vi "Add file.vi"(8 "error in (no error)":errorcluster, 9 "Insert in front":bool, 10 "File Path":path, 11 "MagLabGraph in":refnum<class "XY Plot.lvclass">) -> (0 "error out":errorcluster, 2 "Success":bool, 3 "MagLabGraph out":refnum<class "XY Plot.lvclass">)   [LabVIEW 2019, in "XY Plot.lvclass"]
uses:
  XY Plot.lvclass
  C:/Program Files/National Instruments/LabVIEW 2019/vi.lib/ActorFramework/Actor/Actor.lvclass
  C:/GitHub/LabActor/Plots/Plot/Plot.lvclass
  <vilib>/ActorFramework/Actor/Actor.lvclass/Actor.ctl
  <vilib>/ActorFramework/Message Enqueuer/Message Enqueuer.lvclass/Message Enqueuer.ctl
  Plot Messages/Add file Msg/Add file Msg.lvclass/Add file Msg.ctl
  XY Plot.lvclass/XY Plot.ctl
  Plot/Plot.lvclass/Plot.ctl
  Read File-group-channel.vi
  Plot/Read File history depth.vi
  <vilib>/ActorFramework/Message Enqueuer/Init from Existing Queue.vi
  Plot Messages/Add file Msg/Add file Msg.lvclass
  C:/Program Files/National Instruments/LabVIEW 2019/vi.lib/ActorFramework/Message/Message.lvclass
  <vilib>/ActorFramework/Time-Delayed Send Message/Time-Delayed Send Message.vi
  Plot/Plot.lvclass
  <vilib>/ActorFramework/Message Enqueuer/Message Enqueuer.lvclass
  <vilib>/ActorFramework/Actor/Actor.lvclass
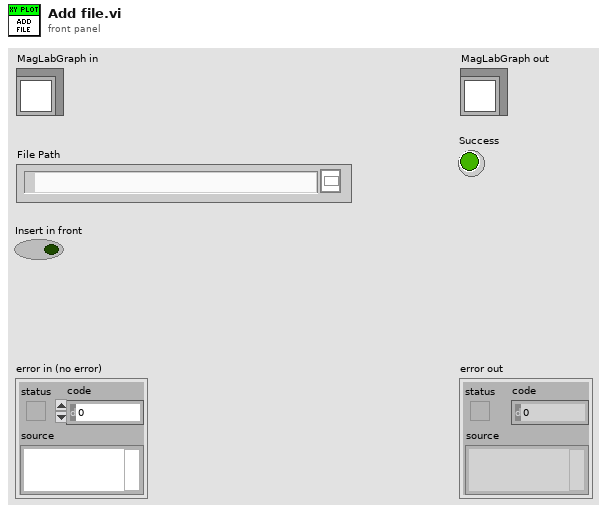
[diagram p1: front panel]
types:
  T1 = cluster{"File Path Control":path, "Group":string, "Channel":string, "Abbreviated":string}[]
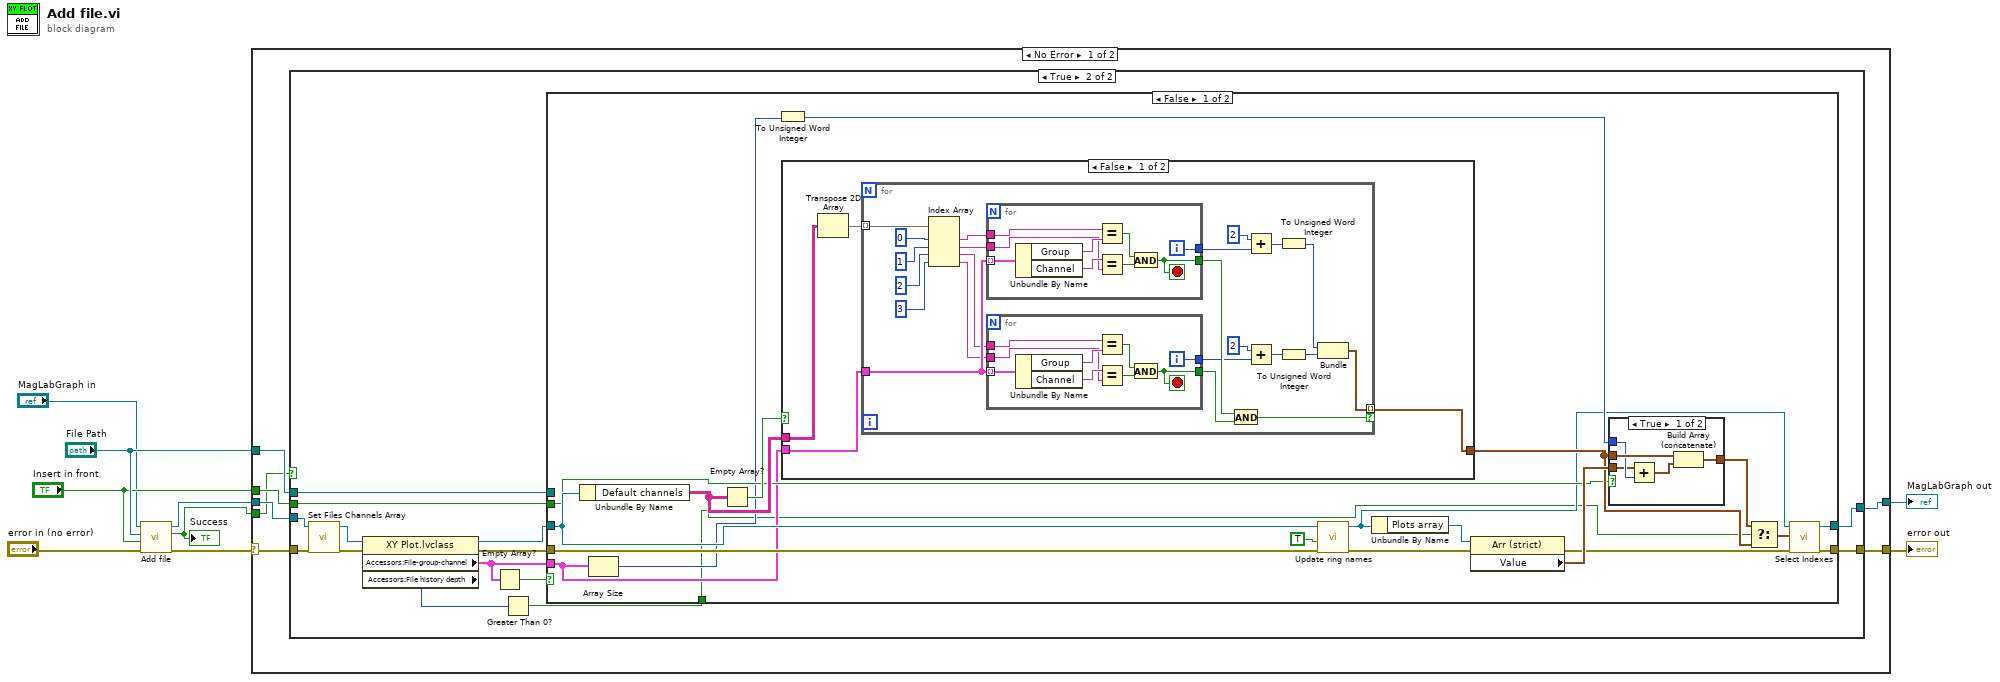
[diagram p0: block diagram]
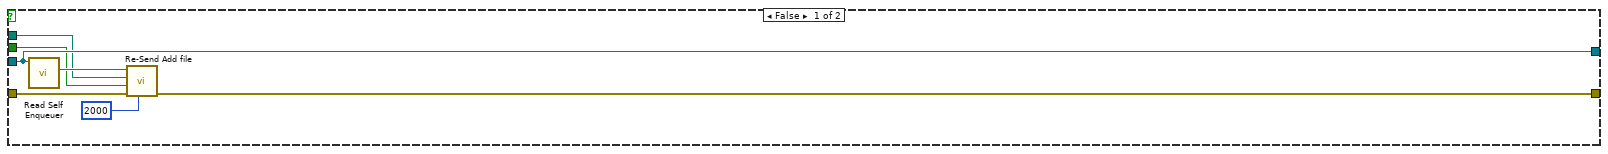
[diagram p2: hidden frame]
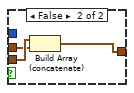
[diagram p3: hidden frame]
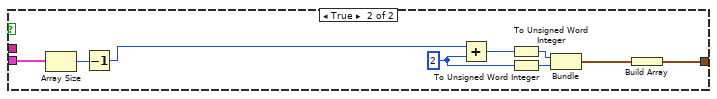
[diagram p4: hidden frame]
diagram:
  n1 = call-parent "Add file.vi"("error in (no error)"="error in (no error)", "Insert in front"="Insert in front", "File Path"="File Path", "Plot in"="MagLabGraph in") -> ("error out"=w6:errorcluster, "Success"=w3:bool, "Plot out"=w1:refnum<class "XY Plot.lvclass">)  [unwired: 5 in]
  "Success" <- w3
  n2 = case shown="No Error" w6 {
    selector: w6 -> [w11 w122]
    tunnel: [w14 w122] -> w7
    tunnel: [w15 w121] -> w8
    tunnel: w1 -> [w16 w121]
    tunnel: "File Path" -> [w13 _]
    tunnel: "Insert in front" -> [w12 _]
    tunnel: w3 -> [w10 _]
    frame No Error {
      n3 = case shown="True" w10 {
        tunnel: w11 -> [w22 w28]
        tunnel: w16 -> [w20 w37]
        tunnel: [w20 w36] -> w15
        tunnel: [w21 w35] -> w14
        tunnel: w13 -> [w19 w34]
        tunnel: w12 -> [w18 w26]
        frame False {
          n4 = call <vilib>:"Read Self Enqueuer.vi"("Actor"=w20) -> ("Self Enqueuer"=w23:refnum<class "Message Enqueuer.lvclass">)  [unwired: 10 in]
          n5 = call "Re-Send Add file.vi"("Milliseconds To Wait"=2000, "error in (no error)"=w22, "Insert in front"=w18, "File Path Control"=w19, "Message Enqueuer"=w23) -> ("error out"=w21:errorcluster)  [unwired: 5 in, 1 out]
        }
        frame True {
          n6 = call-dynamic "Set Files Channels Array.vi"("error in (no error)"=w28, "Plot in"=w37) -> ("error out"=w30:errorcluster, "Plot out"=w32:refnum<class "XY Plot.lvclass">)  [unwired: 8 in]
          n7 = property class="XY Plot.lvclass"(reference=w32, error in=w30) -> (reference out=w31:refnum<class "XY Plot.lvclass">, error out=w27:errorcluster, "Accessors:File-group-channel"=w29:T1, "Accessors:File history depth"=w25:i32)
          n8 = Empty Array?(array=w29) -> (empty?=w33:bool)
          n9 = Greater Than 0?(x=w25) -> (x > 0?=w24:bool)
          n10 = case shown="False" w33 {
            tunnel: w31 -> [w57 w119]
            tunnel: [w42 w119] -> w36
            tunnel: w29 -> [w46 _]
            tunnel: [w40 w120] -> w35
            tunnel: w26 -> [w47 _]
            tunnel: w34 -> [_ _]
            tunnel: w27 -> [w52 w120]
            tunnel: w24 -> [w38 _]
            frame False {
              n11 = Unbundle By Name(w57) -> ("Default channels"=w50:string[][])
              n12 = Array Size(array=w46) -> (size(s)=w45:i32)
              n13 = Empty Array?(array=w50) -> (empty?=w51:bool)
              n14 = To Unsigned Word Integer(number=w45) -> (unsigned 16bit integer=w44:u16)
              n15 = case shown="False" w51 {
                tunnel: w46 -> [w66 w111]
                tunnel: [w67 w112] -> w48
                tunnel: w50 -> [w69 _]
                frame False {
                  n16 = Transpose 2D Array(2D array=w69) -> (transposed array=w68:string[][])
                  n17 = for {
                    tunnel: w68 -> [w91] mode=indexing
                    tunnel: w66 -> [w84]
                    tunnel: [w77] -> w67 mode=indexing if=w76
                    n18 = Index Array(array=w91, index #1=0 ("index"), index #2=1 ("index"), index #3=2 ("index"), index #4=3 ("index")) -> (element #1=w86:string, element #2=w85:string, element #3=w83:string, element #4=w82:string)
                    n19 = for {
                      tunnel: w84 -> [w109] mode=indexing
                      tunnel: w86 -> [w107]
                      tunnel: w85 -> [w105]
                      tunnel: [w102] -> w81
                      tunnel: [w101] -> w74
                      i -> [w101]
                      stop <- w102 stop-if-true
                      n20 = Unbundle By Name(w109) -> ("Group"=w108:string, "Channel"=w106:string)
                      n21 = Equal?(x=w107, y=w108) -> (x = y?=w103:bool)
                      n22 = Equal?(x=w106, y=w105) -> (x = y?=w104:bool)
                      n23 = And(x=w103, y=w104) -> (x .and. y?=w102:bool)
                    }
                    n24 = for {
                      tunnel: w84 -> [w100] mode=indexing
                      tunnel: w83 -> [w98]
                      tunnel: w82 -> [w96]
                      tunnel: [w93] -> w80
                      tunnel: [w92] -> w71
                      i -> [w92]
                      stop <- w93 stop-if-true
                      n25 = Unbundle By Name(w100) -> ("Group"=w99:string, "Channel"=w97:string)
                      n26 = Equal?(x=w98, y=w99) -> (x = y?=w94:bool)
                      n27 = Equal?(x=w97, y=w96) -> (x = y?=w95:bool)
                      n28 = And(x=w94, y=w95) -> (x .and. y?=w93:bool)
                    }
                    n29 = And(x=w81, y=w80) -> (x .and. y?=w76:bool)
                    n30 = Add(x=2, y=w74) -> (x+y=w73:i32)
                    n31 = Add(x=2, y=w71) -> (x+y=w70:i32)
                    n32 = To Unsigned Word Integer(number=w73) -> (unsigned 16bit integer=w79:u16)
                    n33 = To Unsigned Word Integer(number=w70) -> (unsigned 16bit integer=w78:u16)
                    n34 = Bundle(w79, w78) -> (w77:cluster{u16, u16})  [unwired: 1 in]
                  }
                }
                frame True {
                  w110 = 2 ("x")
                  n35 = Array Size(array=w111) -> (size(s)=w116:i32)
                  n36 = Decrement(x=w116) -> (x-1=w114:i32)
                  n37 = Add(x=w114, y=w110) -> (x+y=w113:i32)
                  n38 = To Unsigned Word Integer(number=w113) -> (unsigned 16bit integer=w117:u16)
                  n39 = To Unsigned Word Integer(number=w110) -> (unsigned 16bit integer=w115:u16)
                  n40 = Bundle(w117, w115) -> (w118:cluster{u16, u16})  [unwired: 1 in]
                  n41 = Build Array(w118) -> (w112:cluster{u16, u16}[])
                }
              }
              n42 = call "Update ring names.vi"("error in (no error)"=w52, "Update from File-group-channel"=TRUE, "MagLabGraph in"=w57) -> ("error out"=w55:errorcluster, "MagLabGraph out"=w43:refnum<class "XY Plot.lvclass">)  [unwired: 7 in]
              n43 = Unbundle By Name(w43) -> ("Plots array"=w56:refnum<vi>)
              n44 = property class="Arr (strict)"(reference=w56, error in=w55) -> (error out=w39:errorcluster, "Value"=w54:cluster{"X":u16, "Y":u16}[])  [unwired: 1 out]
              n45 = case shown="True" w47 {
                tunnel: w54 -> [w58 w64]
                tunnel: [w62 w65] -> w49
                tunnel: w48 -> [w61 w63]
                tunnel: w44 -> [w60 _]
                frame True {
                  n46 = Add(x=w58, y=w60) -> (x+y=w59:cluster{"X":u16, "Y":u16}[])
                  n47 = Build Array (concatenate)(w61, w59) -> (w62:cluster{"X":u16, "Y":u16}[])
                }
                frame False {
                  n48 = Build Array (concatenate)(w64, w63) -> (w65:cluster{"X":u16, "Y":u16}[])
                }
              }
              n49 = Select(t=w49, s=w38, f=w48) -> (s? t:f=w41:cluster{"X":u16, "Y":u16}[])
              n50 = call-dynamic "Select Indexes.vi"("error in (no error)"=w39, "Plot Indexes Array"=w41, "MagLabGraph in"=w43) -> ("error out"=w40:errorcluster, "MagLabGraph out"=w42:refnum<class "XY Plot.lvclass">)  [unwired: 7 in]
            }
            frame True {
            }
          }
        }
      }
    }
    frame Error {
    }
  }
  "error out" <- w7
  "MagLabGraph out" <- w8
